vi "PiezoStart.vi"(2 "WAVE":T1={"Speed"=0.0, "Stiffness (0.95)"=0.95, "Linear Stroke"=0.0, "Delay"=0.0} {"Delay" format="%.2f"; "Linear Stroke" format="%.2f"; "Stiffness (0.95)" format="%.2f"; "Speed" format="%.2f"}, 9 "error in (no error)":errorcluster caption="entrée d'erreur") -> (6 "error out":errorcluster caption="sortie d'erreur")   [LabVIEW 2009]
uses:
  Controls/PIEZO.WAVE.ctl
  Controls/PIEZO.STATE.ctl
  Controls/PIEZO.COMMAND.ctl
  Controls/PIEZO.COMMANDBASIC.ctl
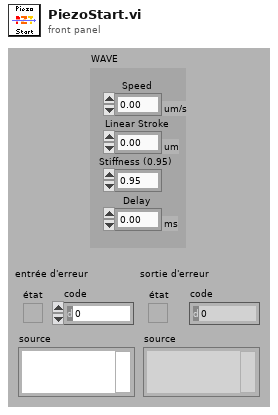
[diagram p1: front panel]
types:
  T1 = typedef "PIEZO.WAVE.ctl" = cluster{"Speed":dbl[unit], "Stiffness (0.95)":dbl, "Linear Stroke":dbl[unit], "Delay":dbl[unit]}
  T2 = typedef "PIEZO.STATE.ctl" = enum16{"IDLE", "STARTING", "RUNNING", "STOPPING", "OFF"}
  T3 = typedef "PIEZO.COMMAND.ctl" = cluster{"Command":T4, "WAVE":T1}
  T4 = typedef "PIEZO.COMMANDBASIC.ctl" = enum16{"RUN", "STOP", "QUIT"}
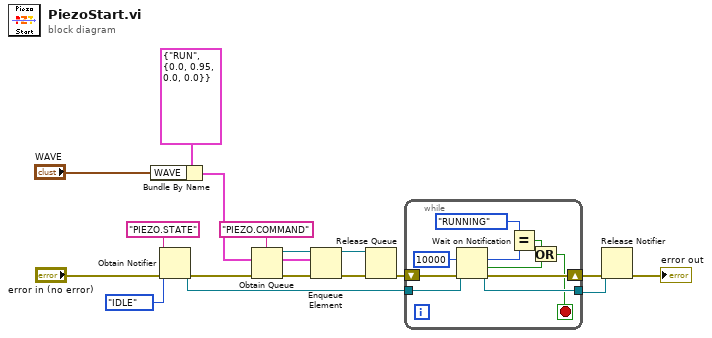
[diagram p0: block diagram]
diagram:
  n1 = Bundle By Name(cluster=T3 {"Command"=enum."RUN", "WAVE"={"Speed"=0.0, "Stiffness (0.95)"=0.95, "Linear Stroke"=0.0, "Delay"=0.0}} ("COMMAND"), "WAVE"="WAVE") -> (w10:T3)
  n2 = Obtain Notifier(name (unnamed)="PIEZO.STATE" ("nom (aucun)"), notification data type=PIEZO.STATE."IDLE" ("STATE"), error in (no error)="error in (no error)") -> (notifier out=w4:refnum<notifier>, error out=w8:errorcluster)  [unwired: 1 in, 1 out]
  n3 = Obtain Queue(name (unnamed)="PIEZO.COMMAND" ("nom (aucun)"), element data type=w10, error in (no error)=w8) -> (queue out=w13:refnum<queue>, error out=w14:errorcluster)  [unwired: 2 in, 1 out]
  n4 = Enqueue Element(queue=w13, element=w10, error in (no error)=w14) -> (queue out=w12:refnum<queue>, error out=w11:errorcluster)  [unwired: 1 in, 1 out]
  n5 = Release Queue(queue=w12, error in (no error)=w11) -> (error out=w5:errorcluster)  [unwired: 1 in, 2 out]
  n6 = while {
    tunnel: w4 -> [w25]
    shift-right: [w26] -> w3
    shift-left: w5 -> [w27]
    tunnel: [w24] -> w2
    stop <- w18 stop-if-true
    n7 = Wait on Notification(notifier=w25, timeout in ms (-1)=10000 ("timeout en ms (-1)"), error in (no error)=w27) -> (notifier out=w24:refnum<notifier>, notification=w22:T2, timed out?=w19:bool, error out=w26:errorcluster)  [unwired: 1 in]
    n8 = Equal?(x=PIEZO.STATE."RUNNING" ("notification"), y=w22) -> (x = y?=w20:bool)
    n9 = Or(x=w20, y=w19) -> (x .or. y?=w18:bool)
  }
  n10 = Release Notifier(notifier=w2, error in (no error)=w3) -> (error out=→"error out":errorcluster)  [unwired: 1 in, 2 out]
